vi "replaceNameInXMLStringWithDesiredName.vi"(8 "error in":errorcluster, 11 "xmlString":string) -> (0 "error out":errorcluster, 3 "revisedXMLString":string)   [LabVIEW 2016, in "UnitsAndXML.lvlib"]
uses:
  <userlib>/Common/UnitsAndXML/UnitsAndXML.lvlib
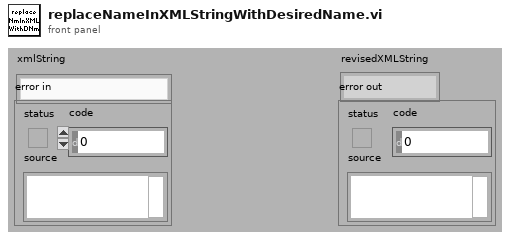
[diagram p1: front panel]
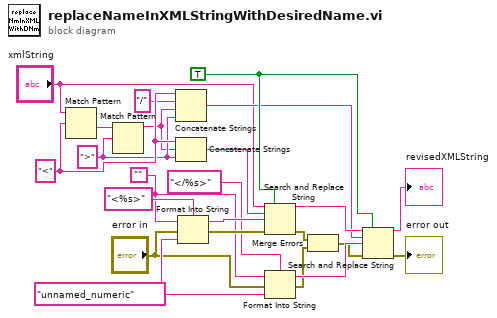
[diagram p0: block diagram]
diagram:
  w1 = ""
  w7 = "unnamed_numeric" ("Name")
  w13 = ">" ("regular expression")
  w15 = "<" ("regular expression")
  w19 = TRUE ("replace all? (F)")
  n1 = Match Pattern(string="xmlString", regular expression=w15) -> (after substring=w14:string)  [unwired: 1 in, 3 out]
  n2 = Match Pattern(string=w14, regular expression=w13) -> (before substring=w12:string)  [unwired: 1 in, 3 out]
  n3 = Concatenate Strings(w15, "/" ("string"), w12, w13) -> (w17:string)
  n4 = Concatenate Strings(w15, w12, w13) -> (w18:string)
  n5 = Format Into String(format string="<%s>" ("search string"), initial string=w1, error in="error in", w7) -> (resulting string=w22:string, error out=w23:errorcluster)
  n6 = Search and Replace String(replace all?=w19, input string="xmlString", search string=w18, replace string=w22, error in=w23) -> (result string=w20:string, error out=w5:errorcluster)  [unwired: 3 in, 2 out]
  n7 = Format Into String(format string="</%s>" ("search string"), initial string=w1, error in="error in", w7) -> (resulting string=w21:string, error out=w4:errorcluster)
  n8 = Merge Errors(w5, w4) -> (w3:errorcluster)
  n9 = Search and Replace String(replace all?=w19, input string=w20, search string=w17, replace string=w21, error in=w3) -> (result string=→"revisedXMLString":string, error out=→"error out":errorcluster)  [unwired: 3 in, 2 out]
